vi "DipeshBoard.vi"() -> ()   [LabVIEW 2016]
uses:
  VIs/uPythonX/uPythonX.xctl
panel:
  in  "AccuWeather":T1(xcontrol)={"VISA Refnum in"="ASRL42::INSTR", "Python Code"="import machine, network, ujson, urequests, utime\nfrom pyb import LED\n\nWiFi = network.WLAN()\nled = LED(1) # 1=red, 2=green, 3=blue\n\ndef connect():\n     if not WiFi.isconnected():\n          print (\"Connecting ..\")\n          WiFi.active(True)\n          WiFi.connect(\"username\",\"password\")\n          LED(2).on()\n\n          i=0\n          while i < 25 and not WiFi.isconnected():\n               utime.sleep_ms(200)\n               i=i+1\n          if WiFi.isconnected():\n               print (\"Connection succeeded\")\n          else:\n               print (\"Connection failed\")\n\nwhile True:\n     connect()\n     print (\"WiFi: \",WiFi.isconnected())\n     if WiFi.isconnected():\n          LED(2).off()\n          break\n     else:\n          LED(2).on()\n\n# Accuweather\n\nKey = \"Type Key Here\"\n\nurlBase = \"http://dataservice.accuweather.com/currentconditions/v1\"\n\nheaders = {\"Accept\":\"application/json\"}\n\ndef Get():\n     urlValue = urlBase + '/348735?apikey=' + Key + \"&details=true\"\n     try:\n          response = urequests.get(urlValue,headers=headers)\n          value = response.text\n          response.close()\n          data = ujson.loads(value)[0]\n          result = data.get('RelativeHumidity')\n          print(data.get('Temperature').get('Metric').get('Value'))\n          print(data.get('Wind').get('Direction').get('Degrees'))\n          print(data.get('Wind').get('Speed').get('Metric').get('Value'))\n          print(data.get('Pressure').get('Metric').get('Value'))\n   except:\n          print('error')\n          result = 'error'\n     return result\n\nprint (Get())"}
  in  "Motor Control":T1(xcontrol)={"VISA Refnum in"="ASRL42::INSTR", "Python Code"="'''\n1. LED pins: X5 and Y11 \n2. Stand by: W29 \n3. A2in A1in PWMA: W24, W22, W16 \n4. B2in B1in PWMB: W32, W30, Y12 \n5. SCL, SDA: Y9, Y10 (I2C(2))\n7. TX, RX: Y9, Y10 (UART(3))\n8. Servo: X4 (Note: X6 does not work) \n9. TACHO: Y1, Y2 and Y3, Y4\n10. Grove I2C: Y9 (SCL) Y10 (SDA)\n11. Grove Analog: X1 \n12. Pins that connected to the breadboard:\nX1, X2, X3 (mistake in Silkscreen says Y3 but is actually X3), \nX4, X6 (Pins X1-X4 can be used to control Servos) \nY6, Y7, Y8, Y9, Y10 \n\n13. Vcc and Ground headers (on the sides)\n'''\nimport pyb\n\nblue = pyb.Pin('X5', pyb.Pin.OUT)\nyellow = pyb.Pin('Y11', pyb.Pin.OUT)\n\nyellow.value(1)\nblue.value(1)\n\n"}
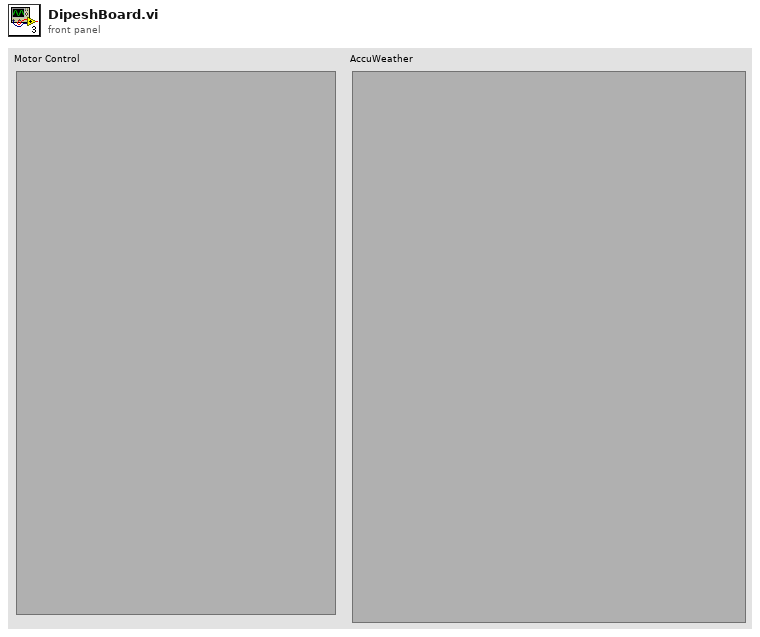
[diagram p1: front panel]
types:
  T1 = cluster{"VISA Refnum in":refnum<visa-resource-name>, "Python Code":string}
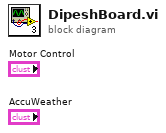
[diagram p0: block diagram]
diagram:
